vi "SP Read Array.vi"(8 "error in":errorcluster, 11 "Temperature Setpoint in":refnum<class "Temperature Setpoint.lvclass">) -> (0 "error out":errorcluster, 1 "Changed or First Call?":bool, 2 "Current Setpoint":dbl[](array[numeric]), 3 "Temperature Setpoint out":refnum<class "Temperature Setpoint.lvclass">)   [LabVIEW 2023, in "Temperature Setpoint.lvclass"]
uses:
  Temperature Setpoint.lvclass
  Temperature Setpoint.lvclass/Temperature Setpoint.ctl
  Parents/Setpoint/Setpoint.lvclass
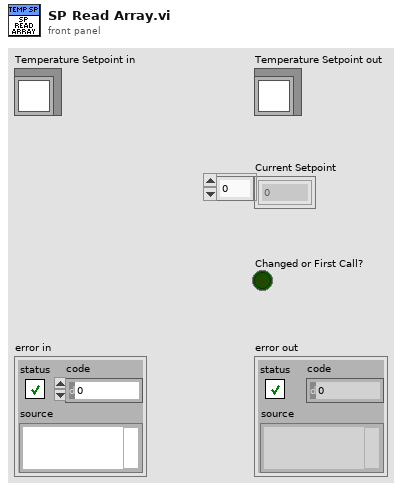
[diagram p1: front panel]
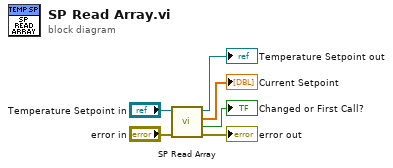
[diagram p0: block diagram]
diagram:
  n1 = call-parent "SP Read Array.vi"("error in"="error in", "Setpoint in"="Temperature Setpoint in") -> ("error out"=→"error out":errorcluster, "Changed or First Call?"=→"Changed or First Call?":bool, "Current Setpoint"=→"Current Setpoint":dbl[], "Setpoint out"=→"Temperature Setpoint out":refnum<class "Temperature Setpoint.lvclass">)  [unwired: 6 in]
